vi "Add Item to Tree.vi"(8 "error in (no error)":errorcluster, 10 "Standard VI Type in":refnum<class "Standard VI Type.lvclass">, 11 "Tree Ref in":refnum<vi>) -> (0 "error out":errorcluster, 1 "Added Tag":string, 2 "Standard VI Type out":refnum<class "Standard VI Type.lvclass">, 3 "Tree Ref out":refnum<vi>)   [LabVIEW 2020, in "Peek Window.lvlib" / "Standard VI Type.lvclass"]
uses:
  Standard VI Type.lvclass
  Symbols Enum.ctl
  Standard VI Type.lvclass/Standard VI Type.ctl
  Peek Window.lvlib
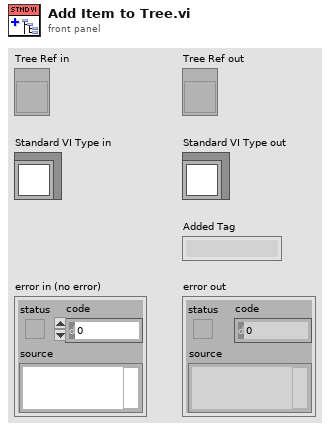
[diagram p1: front panel]
types:
  T1 = typedef "Peek Window.lvlib/Symbols Enum.ctl" = enum16{"<Blank>", "Implementation Mark", "Standard VI", "Dynamic Dispatch VI", "Malleable VI", "Polymorphic VI", "Missing VI", "Express VI"}
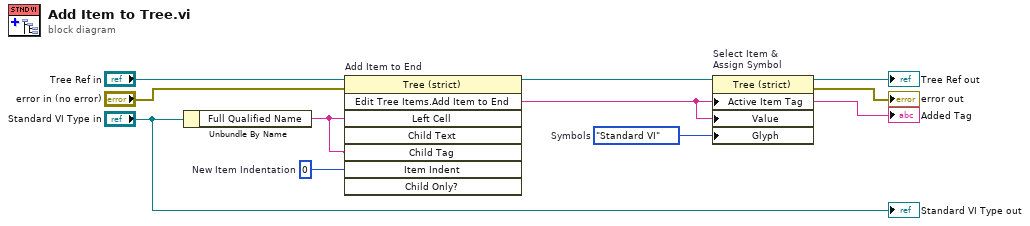
[diagram p0: block diagram]
diagram:
  w6 = Symbols_Enum."Standard VI"  # Symbols
  w8 = 0  # New Item Indentation
  n1 = Unbundle By Name("Standard VI Type in") -> ("Full Qualified Name"=w1:string)
  n2 = invoke on="Add Item to End" class="Tree (strict)" method="Edit Tree Items.Add Item to End"(reference="Tree Ref in", error in="error in (no error)", "Left Cell"=w1, "Child Tag"=w1, "Item Indent"=w8) -> (reference out=w5:refnum<vi>, "Edit Tree Items:Add Item to End"=w2:string)  [unwired: 3 in, 6 out]
  "Added Tag" <- w2
  n3 = property on="Select Item &\nAssign Symbol" class="Tree (strict)"(reference=w5, "Active Item Tag"=w2, "Value"=w2, "Glyph"=w6) -> (reference out=→"Tree Ref out":refnum<vi>, error out=→"error out":errorcluster)  [unwired: 1 in]
  "Standard VI Type out" <- "Standard VI Type in"
